vi "DOE States.vi"(0 "Disable Barometric Pressure":bool, 4 "Enable RMC Collection":bool, 5 "Disable Gas Data":bool, 6 "Disable Temp/Humidity":bool, 7 "Disable Power":bool, 8 "Disable Analog Data":bool, 9 "Disable Flow Rates":bool, 10 "Disable Scale Data":bool, 11 "Scale Disabled Config":bool) -> (3 "States":string)   [LabVIEW 2019]
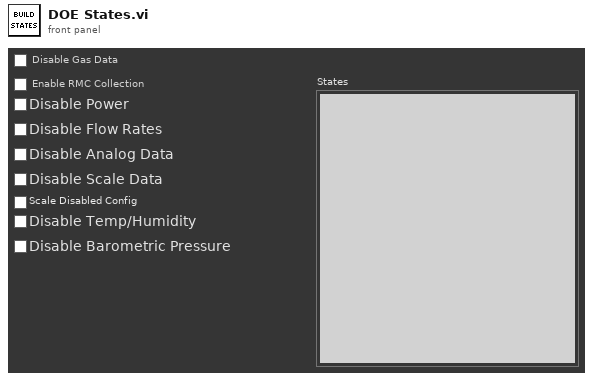
[diagram p1: front panel]
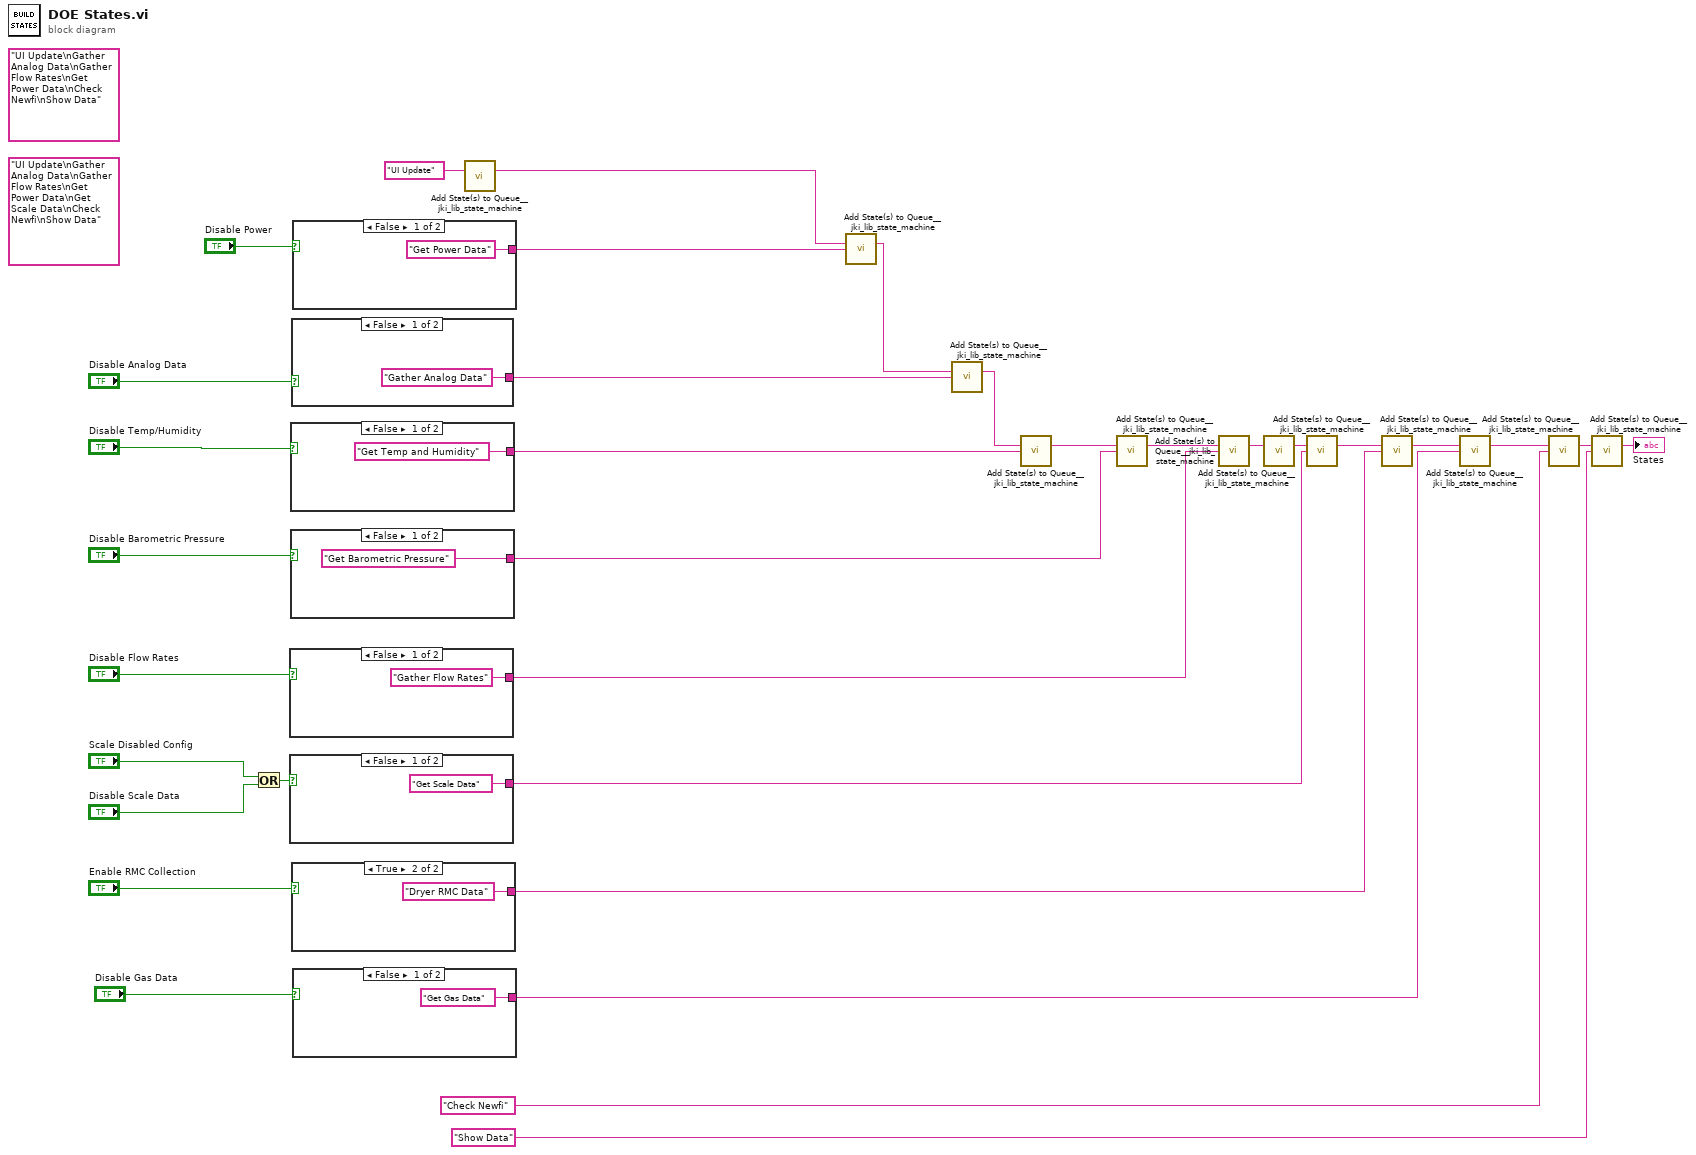
[diagram p0: block diagram]
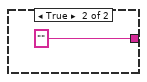
[diagram p2: hidden frame]
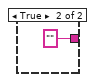
[diagram p3: hidden frame]
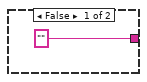
[diagram p4: hidden frame]
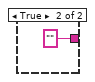
[diagram p5: hidden frame]
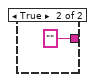
[diagram p6: hidden frame]
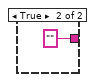
[diagram p7: hidden frame]
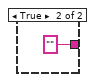
[diagram p8: hidden frame]
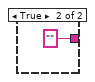
[diagram p9: hidden frame]
diagram:
  (unwired) "UI Update\nGather Analog Data\nGather Flow Rates\nGet Power Data\nCheck Newfi\nShow Data"
  (unwired) "UI Update\nGather Analog Data\nGather Flow Rates\nGet Power Data\nGet Scale Data\nCheck Newfi\nShow Data"
  n1 = Or(x="Scale Disabled Config", y="Disable Scale Data") -> (x .or. y?=w22:bool)
  n2 = case shown="False" "Disable Flow Rates" {
    tunnel: ["Gather Flow Rates" ""] -> w31
    frame False {
    }
    frame True {
    }
  }
  n3 = case shown="False" w22 {
    tunnel: ["Get Scale Data" ""] -> w28
    frame False {
    }
    frame True {
    }
  }
  n4 = case shown="False" "Disable Temp/Humidity" {
    tunnel: ["Get Temp and Humidity" ""] -> w15
    frame False {
    }
    frame True {
    }
  }
  n5 = case shown="False" "Disable Barometric Pressure" {
    tunnel: ["Get Barometric Pressure" ""] -> w6
    frame False {
    }
    frame True {
    }
  }
  n6 = case shown="False" "Disable Analog Data" {
    tunnel: ["Gather Analog Data" ""] -> w32
    frame False {
    }
    frame True {
    }
  }
  n7 = case shown="True" "Enable RMC Collection" {
    tunnel: ["" "Dryer RMC Data"] -> w9
    frame False {
    }
    frame True {
    }
  }
  n8 = case shown="False" "Disable Power" {
    tunnel: ["Get Power Data" ""] -> w13
    frame False {
    }
    frame True {
    }
  }
  n9 = case shown="False" "Disable Gas Data" {
    tunnel: ["Get Gas Data" ""] -> w1
    frame False {
    }
    frame True {
    }
  }
  n10 = call <vilib>:"Add State(s) to Queue__jki_lib_state_machine.vi"("State(s) in (\"\")"="UI Update") -> ("States Out"=w14:string)  [unwired: 14 in]
  n11 = call <vilib>:"Add State(s) to Queue__jki_lib_state_machine.vi"("State(s) in (\"\")"=w14, "State(s) at Back (\"\")"=w13) -> ("States Out"=w12:string)  [unwired: 13 in]
  n12 = call <vilib>:"Add State(s) to Queue__jki_lib_state_machine.vi"("State(s) in (\"\")"=w12, "State(s) at Back (\"\")"=w32) -> ("States Out"=w16:string)  [unwired: 13 in]
  n13 = call <vilib>:"Add State(s) to Queue__jki_lib_state_machine.vi"("State(s) in (\"\")"=w16, "State(s) at Back (\"\")"=w15) -> ("States Out"=w8:string)  [unwired: 13 in]
  n14 = call <vilib>:"Add State(s) to Queue__jki_lib_state_machine.vi"("State(s) in (\"\")"=w8, "State(s) at Back (\"\")"=w6) -> ("States Out"=w7:string)  [unwired: 13 in]
  n15 = call <vilib>:"Add State(s) to Queue__jki_lib_state_machine.vi"("State(s) in (\"\")"=w7, "State(s) at Back (\"\")"=w31) -> ("States Out"=w30:string)  [unwired: 13 in]
  n16 = call <vilib>:"Add State(s) to Queue__jki_lib_state_machine.vi"("State(s) in (\"\")"=w30) -> ("States Out"=w29:string)  [unwired: 14 in]
  n17 = call <vilib>:"Add State(s) to Queue__jki_lib_state_machine.vi"("State(s) in (\"\")"=w29, "State(s) at Back (\"\")"=w28) -> ("States Out"=w10:string)  [unwired: 13 in]
  n18 = call <vilib>:"Add State(s) to Queue__jki_lib_state_machine.vi"("State(s) in (\"\")"=w10, "State(s) at Back (\"\")"=w9) -> ("States Out"=w3:string)  [unwired: 13 in]
  n19 = call <vilib>:"Add State(s) to Queue__jki_lib_state_machine.vi"("State(s) in (\"\")"=w3, "State(s) at Back (\"\")"=w1) -> ("States Out"=w2:string)  [unwired: 13 in]
  n20 = call <vilib>:"Add State(s) to Queue__jki_lib_state_machine.vi"("State(s) in (\"\")"=w2, "State(s) at Back (\"\")"="Check Newfi") -> ("States Out"=w26:string)  [unwired: 13 in]
  n21 = call <vilib>:"Add State(s) to Queue__jki_lib_state_machine.vi"("State(s) in (\"\")"=w26, "State(s) at Back (\"\")"="Show Data") -> ("States Out"=→"States":string)  [unwired: 13 in]
